vi "Test Bench v20 - TDMS.vi"() -> ()   [LabVIEW 2022 SP3]
doc: "Use this template to build a producer/consumer design pattern. Use this template when you need to execute a process, such as data analysis, when a data source, such as a triggered acquisition, produces data at an uneven rate and you need to execute the process when the data becomes available."
uses:
  WhiteNoise.ctl
  <vilib>/Utility/error.llb/DialogType.ctl
  <vilib>/Platform/TimedLoop/XDataNode/timing_clust.ctl
  <vilib>/Platform/TimedLoop/XDataNode/nitl_modes.ctl
  <vilib>/Platform/TimedLoop/XDataNode/wakeup.ctl
  <vilib>/measure/maspectr.llb/FFT Spectrum (Mag-Phase) for 1 Chan.vi
  <vilib>/platform/TimedLoop/XDataNode/XDataNode.xnode
  <vilib>/Platform/TimedLoop/XDataNode/XDNodeRunTimeDep.lvlib
  <vilib>/measure/NI_MAPro.lvlib
panel:
  in  "Folder to save file to":path=path "C:/Users/LAV-UFSC-2023/Documents/LAV-TCC/Dados-Experimentos/Dados-Bancada-LABVIEW"
  out "# pending insert":i32
  out "# pending remove":i32
  out "# elements in queue":i32
  out "Processor 2":i32=-2
  out "Iteration Duration":i64
  out "Processor":i32=-2
  out "Accelerometer":waveform(dbl)(graph)
  out "New file path":path
  in  "Log Data":bool
  in  "view":T1={"dB On (F)"=FALSE, "unwrap phase (F)"=TRUE, "convert to degree (F)"=TRUE}
  out "FFT - Phase":cluster{"f0":dbl, "df":dbl, "phase":dbl[]}(graph)
  out "FFT - Magnitude":cluster{"f0":dbl, "df":dbl, "magnitude":dbl[]}(graph)
  out "Signal Output (V)":waveform(dbl)(graph)
  out "Iteration Duration 2":i64
  in  "Enable Output":bool=TRUE
  in  "Signal Output\nControl":enum32{"White Noise", "Harmonic"}(tab)
  in  "White Noise\nParameters":T3={"Seed"=0.0, "Standard Deviation"=2.0, "Reset"=FALSE, "Iterator"=1.0, "Lower Cut-Off"=5.0, "Upper Cut-Off"=350.0} {"Upper Cut-Off" min=5.0 max=350.0 step=10.0; "Lower Cut-Off" min=5.0 max=350.0 step=10.0; "Standard Deviation" min=0.001 max=3.0 step=0.05 format="%0.2p"}
  in  "Hamonic\nParameters":T4={"Waveform Type"=0, "Frequency (Hz)"=10.0, "Amplitude"=0.25} {"Frequency (Hz)" min=5.0 max=350.0 step=10.0 format="%0.2p"; "Waveform Type" items=["Sine Wave", "Triangle Wave", "Square Wave", "Sawtooth Wave"]; "Amplitude" min=0.001 max=0.3 step=0.05 format="%0.2p"}
  in  "stop":bool
  # "Debug Pannel"
  # "Filter"
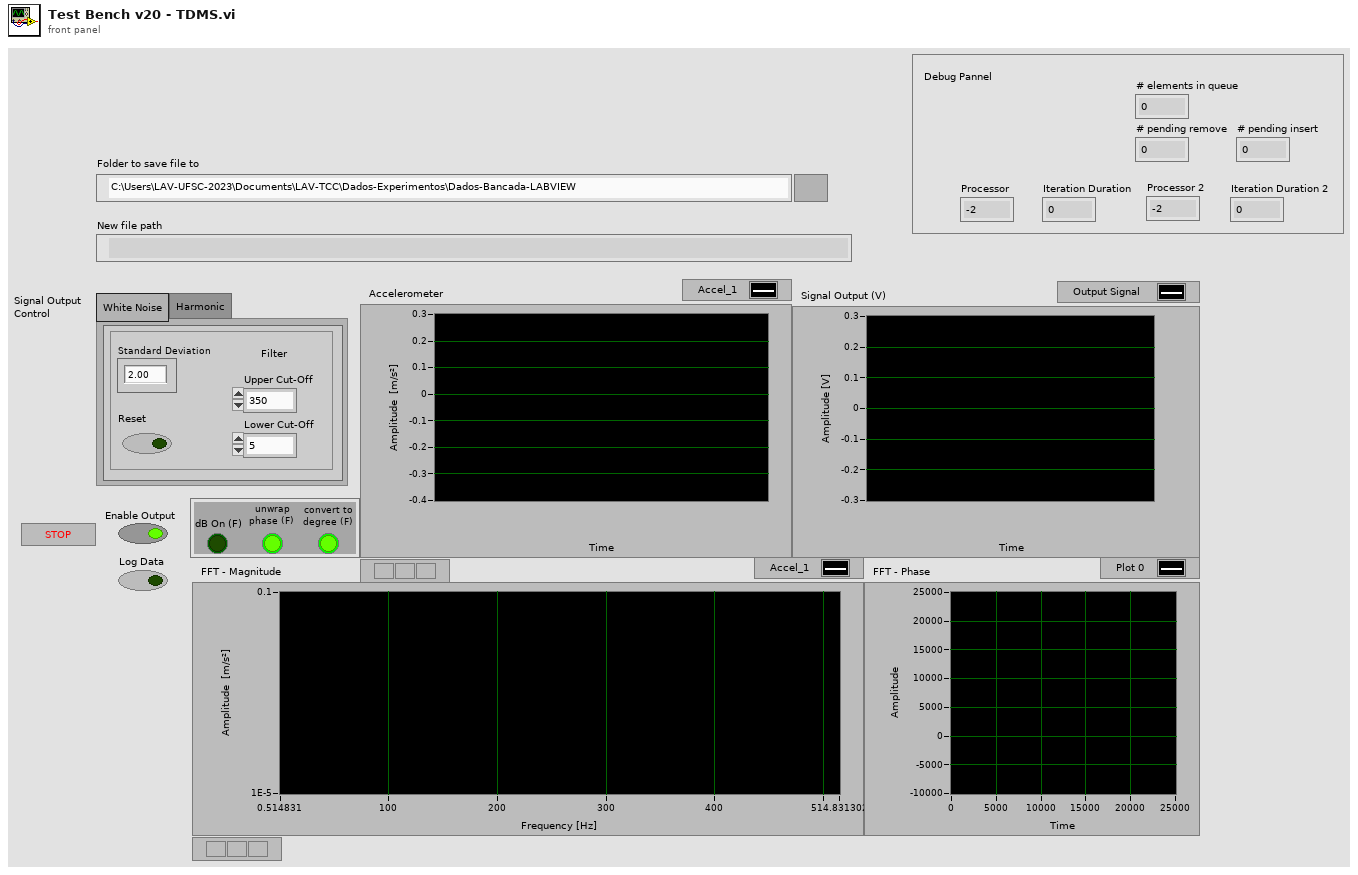
[diagram p1: front panel]
types:
  T1 = cluster{"dB On (F)":bool, "unwrap phase (F)":bool, "convert to degree (F)":bool}
  T2 = typedef "WhiteNoise.ctl" = dbl
  T3 = cluster{"Seed":T2, "Standard Deviation":dbl, "Reset":bool, "Iterator":dbl, "Lower Cut-Off":dbl, "Upper Cut-Off":dbl}
  T4 = cluster{"Waveform Type":u16, "Frequency (Hz)":dbl, "Amplitude":dbl}
  T5 = cluster{"FrameProperties":cluster{"Frame Duration":i64, "Actual Start [i]":i64}, "Accelerometer 1":waveform(dbl), "SignalOut":waveform(dbl)}
  T6 = typedef "DialogType.ctl" = u16
  T7 = typedef "XDNodeRunTimeDep.lvlib/timing_clust.ctl" = cluster{"Expected End [f-1]":u64, "Actual End [f-1]":u64, "Finished Late? [f-1]":bool, "Expected End [i-1]":u64, "Actual End [i-1]":u64, "Finished Late? [i-1]":bool, "Expected Start [i]":u64, "Actual Start [i]":u64, "Expected Start [f]":u64, "Actual Start [f]":u64, "Source Name":string, "Structure Name":string, "Period":i64, "Deadline":i64, "Offset":i64, "Start":i64, "Priority":i32, "Timeout":i32, "Mode":T8, "Wakeup Reason":T9, "Error":errorcluster, "Source Type":string, "Secondary Source Type":string, "Global End Time":u64, "Global Start Time":u64, "Frame Duration":u64, "Iteration Duration":u64, "Assigned CPU":i32, "I/O Scan Engine Mode":u32}
  T8 = typedef "XDNodeRunTimeDep.lvlib/nitl_modes.ctl" = enum32{"No Change", "Process missed periods, maintain original phase", "Discard missed periods, maintain original phase", "Process missed periods, ignore original phase", "Discard missed periods, ignore original phase"}
  T9 = typedef "XDNodeRunTimeDep.lvlib/wakeup.ctl" = enum32{"Normal", "Aborted", "Asynchronous wakeup", "Timing source error", "Timed loop error", "Timeout"}
  T10 = cluster{"Frame Duration":i64, "Actual Start [i]":i64}
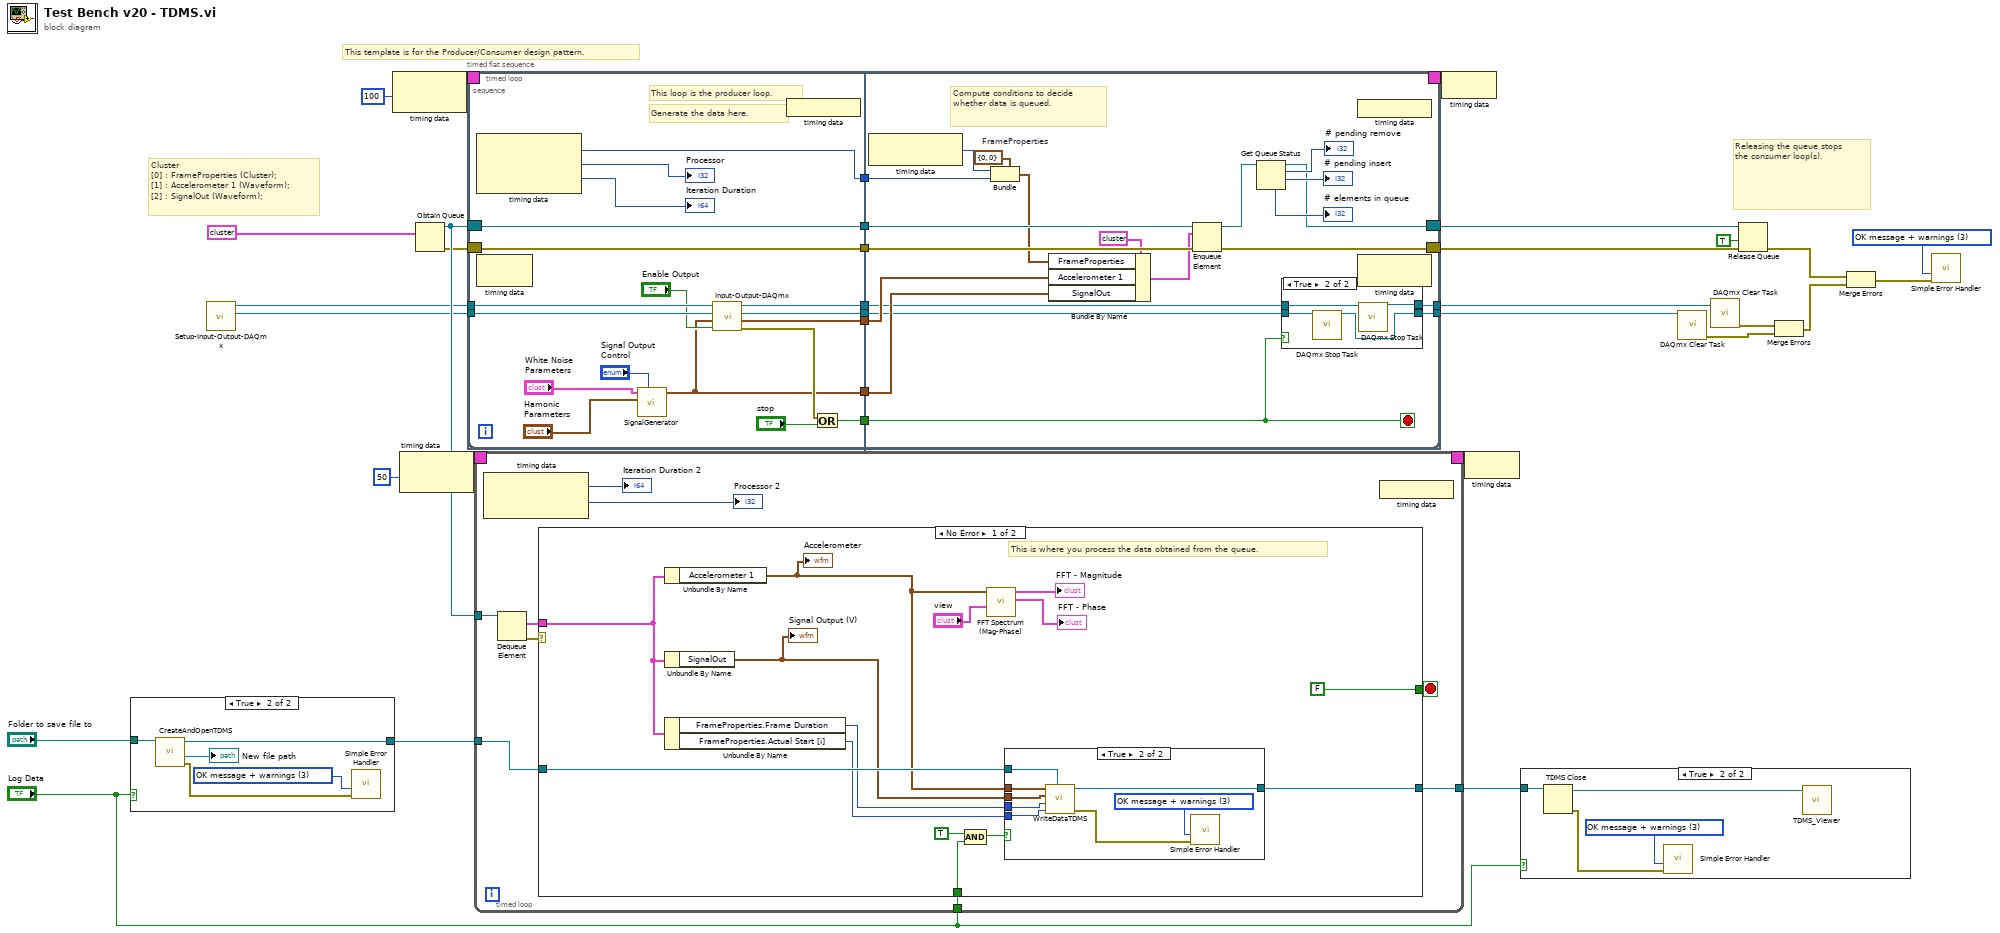
[diagram p0: block diagram]
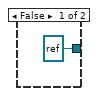
[diagram p3: hidden frame]
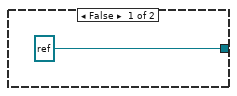
[diagram p4: hidden frame]
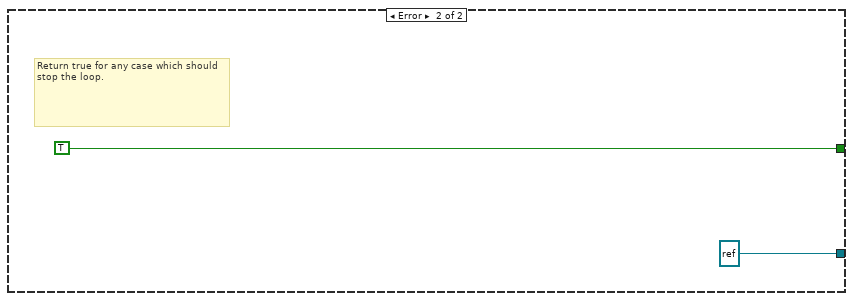
[diagram p5: hidden frame]
diagram:
  w22 = T6 3 items=["no dialog", "OK message", "continue or stop message", "OK message + warnings", "continue/stop + warnings"] ("type of dialog (OK msg:1)")
  # "Cluster\n[0] : FrameProperties (Cluster);\n[1] : Accelerometer 1 (Waveform);\n[2] : SignalOut (Waveform);"
  # "Releasing the queue stops the consumer loop(s)."
  # "This template is for the Producer/Consumer design pattern."
  n1 = case shown="True" "Log Data" {
    tunnel: [refnum<k34> refnum ("tdms file out") w29] -> w10
    tunnel: "Folder to save file to" -> [_ w28]
    frame False {
    }
    frame True {
      w31 = T6 3 items=["no dialog", "OK message", "continue or stop message", "OK message + warnings", "continue/stop + warnings"] ("type of dialog (OK msg:1)")
      n2 = call "CreateAndOpenTDMS.vi"("Folder to save file to"=w28) -> ("error out"=w32:errorcluster, "New file path"=→"New file path":path, "tdms file out"=w29:refnum<k34>)  [unwired: 8 in]
      n3 = call <vilib>:"Simple Error Handler.vi"("type of dialog (OK msg:1)"=w31, "error in (no error)"=w32) -> ()  [unwired: 3 in, 5 out]
    }
  }
  n4 = call "Setup-Input-Output-DAQmx.vi"() -> ("Output task"=w16:refnum<k21>, "Input Task"=w17:refnum<k21>)  [unwired: 9 in, 1 out]
  n5 = node-c288(100 ("Priority")) -> (w15:T7)
  n6 = node-c288(50 ("Priority")) -> (w13:T7)
  n7 = Obtain Queue(element data type=T5 {"FrameProperties"={"Frame Duration"=0, "Actual Start [i]"=0}, "Accelerometer 1"={"t0"=timestamp(0 s since 1904-01-01), "dt"=1.0, "Y"=[]}, "SignalOut"={"t0"=timestamp(0 s since 1904-01-01), "dt"=1.0, "Y"=[]}} ("input cluster")) -> (queue out=w26:refnum<queue>, error out=w25:errorcluster)  [unwired: 4 in, 1 out]
  n8 = timed-loop {
    shift-right: [w37] -> w23
    shift-left: w25 -> [w38]
    shift-right: [w35] -> w24
    shift-left: w26 -> [w36]
    tunnel: [w33] -> w19
    tunnel: [w34] -> w18
    tunnel: w17 -> [w40]
    tunnel: w16 -> [w39]
    timing: w15 -> [_]
    timing-out: [_] -> w14
    stop <- w84 stop-if-true
    n9 = timed-sequence {
      timing: _ -> [_]
      timing-out: _ -> [_]
      tunnel: w40 -> [w56]
      tunnel: w39 -> [w55]
      tunnel: w38 -> [w54]
      tunnel: [w53] -> w37
      tunnel: w36 -> [w52]
      tunnel: [w51] -> w35
      tunnel: [w42] -> w34
      tunnel: [w41] -> w33
      n10 = timed-flat-sequence {
        tunnel: w56 -> [w72]
        tunnel: w55 -> [w71]
        tunnel: w54 -> [w63]
        tunnel: w52 -> [w62]
        tunnel: [w74] -> w50
        tunnel: [w73] -> w49
        tunnel: [w63] -> w48
        tunnel: [w62] -> w47
        tunnel: [w70] -> w46
        tunnel: [w61] -> w45
        tunnel: [w57] -> w44
        tunnel: [w60] -> w43
        tunnel: [w85] -> w51
        tunnel: [w99] -> w53
        tunnel: w50 -> [w82]
        tunnel: w49 -> [w83]
        tunnel: w48 -> [w100]
        tunnel: w47 -> [w98]
        tunnel: w46 -> [w84]
        tunnel: w45 -> [w96]
        tunnel: w44 -> [w95]
        tunnel: w43 -> [w94]
        tunnel: [w81] -> w42
        tunnel: [w80] -> w41
        frame #0 {
          # "Generate the data here."
          # "This loop is the producer loop."
          n11 = node-c288() -> (w61:i64, →"Processor":i32, →"Iteration Duration":i64)  [unwired: 1 in]
          n12 = call "SignalGenerator.vi"("Signal Output\nControl"="Signal Output\nControl", "Hamonic\nParameters"="Hamonic\nParameters", "White Noise\nParameters"="White Noise\nParameters") -> ("Signal Out"=w57:waveform(dbl))  [unwired: 8 in]
          n13 = call "Input-Output-DAQmx.vi"("Enable Output"="Enable Output", "data"=w57, "task/channels in"=w71, "Input Task In"=w72) -> ("error out"=w68:errorcluster, "Input Data Sink"=w60:waveform(dbl), "task out"=w74:refnum<k21>, "Input task Out"=w73:refnum<k21>)  [unwired: 4 in]
          n14 = node-c288() -> ()  [unwired: 1 out]
          n15 = Or(x=w68, y="stop") -> (x .or. y?=w70:bool)
        }
        frame #1 {
          w91 = T10 {"Frame Duration"=0, "Actual Start [i]"=0}  # FrameProperties
          # "Compute conditions to decide whether data is queued."
          n16 = node-c288() -> (w97:i64)  [unwired: 1 in]
          n17 = Bundle(cluster=w91, "Frame Duration"=w97, "Actual Start [i]"=w96) -> (w92:T10)
          n18 = Bundle By Name(cluster=T5 {"FrameProperties"={"Frame Duration"=0, "Actual Start [i]"=0}, "Accelerometer 1"={"t0"=timestamp(0 s since 1904-01-01), "dt"=1.0, "Y"=[]}, "SignalOut"={"t0"=timestamp(0 s since 1904-01-01), "dt"=1.0, "Y"=[]}} ("input cluster"), "FrameProperties"=w92, "Accelerometer 1"=w94, "SignalOut"=w95) -> (w93:T5)
          n19 = Enqueue Element(queue=w98, element=w93, error in (no error)=w100) -> (queue out=w86:refnum<queue>, error out=w99:errorcluster)  [unwired: 1 in, 1 out]
          n20 = Get Queue Status(queue=w86) -> (queue out=w85:refnum<queue>, # pending remove=→"# pending remove":i32, # pending insert=→"# pending insert":i32, # elements in queue=→"# elements in queue":i32)  [unwired: 2 in, 4 out]
          n21 = case shown="True" w84 {
            tunnel: [w101 w106] -> w81
            tunnel: w83 -> [w101 w105]
            tunnel: w82 -> [w102 w104]
            tunnel: [w102 w103] -> w80
            frame False {
            }
            frame True {
              n22 = call <vilib>:"DAQmx Stop Task.vi"("task/channels in"=w104) -> ("task out"=w103:refnum<k21>)  [unwired: 13 in, 1 out]
              n23 = call <vilib>:"DAQmx Stop Task.vi"("task/channels in"=w105) -> ("task out"=w106:refnum<k21>)  [unwired: 13 in, 1 out]
            }
          }
          n24 = node-c288() -> ()  [unwired: 1 out]
        }
      }
    }
    n25 = node-c288() -> ()  [unwired: 1 in, 1 out]
    n26 = node-c288() -> ()  [unwired: 1 in, 1 out]
  }
  n27 = timed-loop {
    tunnel: w26 -> [w120]
    timing: w13 -> [_]
    timing-out: [_] -> w12
    tunnel: w10 -> [w115]
    tunnel: [w114] -> w5
    tunnel: "Log Data" -> [w113]
    stop <- w117 stop-if-true
    n28 = node-c288() -> (→"Iteration Duration 2":i64, →"Processor 2":i32)  [unwired: 1 in]
    n29 = Dequeue Element(queue=w120) -> (element=w118:T5, error out=w119:errorcluster)  [unwired: 2 in, 2 out]
    n30 = case shown="No Error" w119 {
      tunnel: w118 -> [w134 _]
      tunnel: [FALSE TRUE] -> w117
      tunnel: w115 -> [w135 _]
      tunnel: [w129 refnum<k34> refnum ("tdms file out")] -> w114
      tunnel: w113 -> [w126 _]
      frame No Error {
        # "This is where you process the data obtained from the queue."
        n31 = Unbundle By Name(w134) -> ("Accelerometer 1"=w133:waveform(dbl))
        "Accelerometer" <- w133
        n32 = Unbundle By Name(w134) -> ("SignalOut"=w132:waveform(dbl))
        "Signal Output (V)" <- w132
        n33 = Unbundle By Name(w134) -> ("FrameProperties.Frame Duration"=w131:i64, "FrameProperties.Actual Start [i]"=w130:i64)
        n34 = And(x=TRUE, y=w126) -> (x .and. y?=w127:bool)
        n35 = call-poly <vilib>:"FFT Spectrum (Mag-Phase).vi"("view"="view", "time signal"=w133) -> ("phase"=→"FFT - Phase":cluster{"f0":dbl, "df":dbl, "phase":dbl[]}, "magnitude"=→"FFT - Magnitude":cluster{"f0":dbl, "df":dbl, "magnitude":dbl[]})  [unwired: 5 in, 3 out]
        n36 = case shown="True" w127 {
          tunnel: w135 -> [_ w147]
          tunnel: w133 -> [_ w146]
          tunnel: w132 -> [_ w145]
          tunnel: w131 -> [_ w144]
          tunnel: w130 -> [_ w143]
          tunnel: [refnum<k34> refnum ("tdms file out") w142] -> w129
          frame False {
          }
          frame True {
            w141 = T6 3 items=["no dialog", "OK message", "continue or stop message", "OK message + warnings", "continue/stop + warnings"] ("type of dialog (OK msg:1)")
            n37 = call "WriteDataTDMS.vi"("tdms file"=w147, "ActualStart[f]"=w143, "TimeInterval"=w144, "SignalOut"=w145, "Accel."=w146) -> ("error out"=w140:errorcluster, "tdms file out"=w142:refnum<k34>)  [unwired: 5 in]
            n38 = call <vilib>:"Simple Error Handler.vi"("type of dialog (OK msg:1)"=w141, "error in (no error)"=w140) -> ()  [unwired: 3 in, 5 out]
          }
        }
      }
      frame Error {
        # "Return true for any case which should stop the loop."
      }
    }
    n39 = node-c288() -> ()  [unwired: 1 out]
  }
  n40 = node-c288(w14) -> ()
  n41 = node-c288(w12) -> ()
  n42 = case shown="True" "Log Data" {
    tunnel: w5 -> [_ w153]
    frame False {
    }
    frame True {
      w152 = T6 3 items=["no dialog", "OK message", "continue or stop message", "OK message + warnings", "continue/stop + warnings"] ("type of dialog (OK msg:1)")
      n43 = TDMS Close(11:w153) -> (0:w151:errorcluster, 3:w150:path)  [unwired: 1 in]
      n44 = call <vilib>:"Simple Error Handler.vi"("type of dialog (OK msg:1)"=w152, "error in (no error)"=w151) -> ()  [unwired: 3 in, 5 out]
      n45 = call "TDMS_Viewer.vi"("Data Directory"=w150) -> ()  [unwired: 11 in]
    }
  }
  n46 = call <vilib>:"DAQmx Clear Task.vi"("task in"=w19) -> ("error out"=w20:errorcluster)  [unwired: 14 in]
  n47 = call <vilib>:"DAQmx Clear Task.vi"("task in"=w18) -> ("error out"=w21:errorcluster)  [unwired: 14 in]
  n48 = Release Queue(queue=w24, force destroy? (F)=TRUE, error in (no error)=w23) -> (error out=w8:errorcluster)  [unwired: 2 out]
  n49 = Merge Errors(w21, w20) -> (w7:errorcluster)
  n50 = Merge Errors(w8, w7) -> (w9:errorcluster)
  n51 = call <vilib>:"Simple Error Handler.vi"("type of dialog (OK msg:1)"=w22, "error in (no error)"=w9) -> ()  [unwired: 3 in, 5 out]
